vi "Calculate sleeping line length_datumLine.vi"(7 "Datum angle":dbl, 8 "error in (no error)":errorcluster, 9 "Datum origin":cluster{"X":sgl, "Y":sgl} {"Y" format="%.2f"; "X" format="%.2f"}, 10 "Line":T1, 11 "Mouse release \npoint":cluster{"X":dbl, "Y":dbl}) -> (0 "error out":errorcluster, 2 "Angle offset":dbl, 3 "Slanting line\nlength":sgl)   [LabVIEW 2019]
uses:
  <vilib>/vision/NI_Vision_Development_Module.lvlib
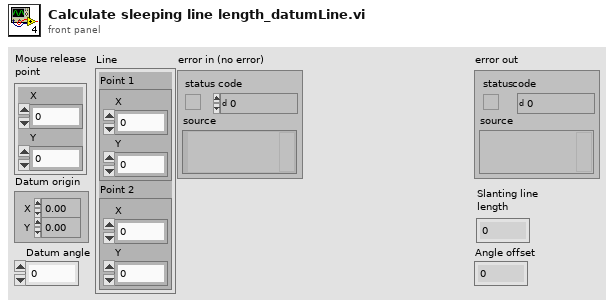
[diagram p1: front panel]
types:
  T1 = cluster{"Point 1":cluster{"X":sgl, "Y":sgl}, "Point 2":cluster{"X":sgl, "Y":sgl}}
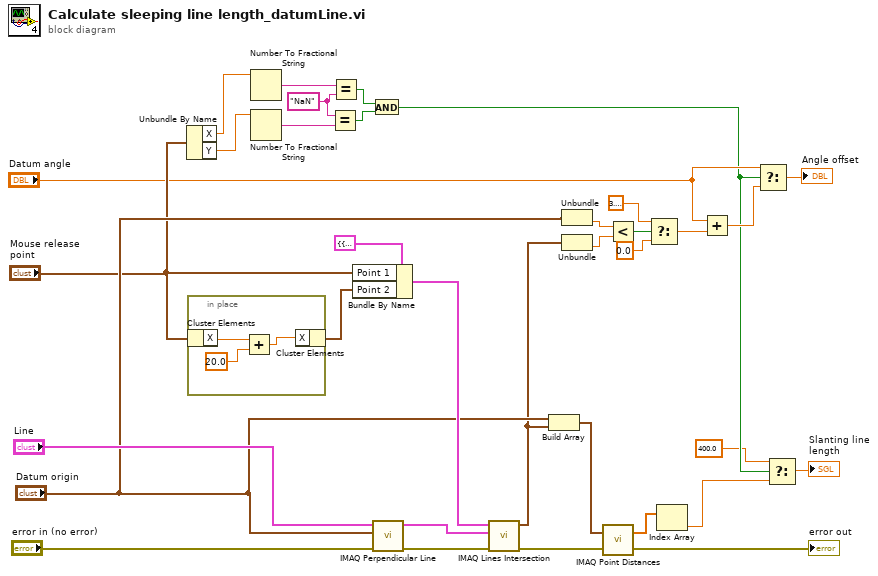
[diagram p0: block diagram]
diagram:
  w10 = "NaN" ("y")
  n1 = Unbundle By Name("Mouse release \npoint") -> ("X"=w14:dbl, "Y"=w13:dbl)
  n2 = in-place {
    n3 = in-place-cluster #1("Mouse release \npoint") -> ("X"=w37:dbl)
    n4 = Add(x=w37, y=20.0) -> (x+y=w35:dbl)
    n5 = in-place-cluster #1("X"=w35) -> (w31:cluster{"X":dbl, "Y":dbl})
  }
  n6 = Number To Fractional String(number=w14) -> (F-format string=w12:string)  [unwired: 3 in]
  n7 = Number To Fractional String(number=w13) -> (F-format string=w11:string)  [unwired: 3 in]
  n8 = Equal?(x=w10, y=w11) -> (x = y?=w8:bool)
  n9 = Equal?(x=w12, y=w10) -> (x = y?=w9:bool)
  n10 = Bundle By Name(cluster=T1 {"Point 1"={"X"=0.0, "Y"=0.0}, "Point 2"={"X"=0.0, "Y"=0.0}} ("Line 1"), "Point 1"="Mouse release \npoint", "Point 2"=w31) -> (w30:T1)
  n11 = And(x=w9, y=w8) -> (x .and. y?=w4:bool)
  n12 = call "IMAQ Perpendicular Line"("error in (no error)"="error in (no error)", "Point"="Datum origin", "Line"="Line") -> ("error out"=w28:errorcluster, "Perpendicular Line"=w29:T1)  [unwired: 6 in, 1 out]
  n13 = call "IMAQ Lines Intersection"("error in (no error)"=w28, "Line 2"=w29, "Line 1"=w30) -> ("error out"=w26:errorcluster, "Intersection Point"=w22:cluster{"X":sgl, "Y":sgl})  [unwired: 6 in, 1 out]
  n14 = Build Array("Datum origin", w22) -> (w27:cluster{"X":sgl, "Y":sgl}[])
  n15 = Unbundle("Datum origin") -> ("Y"=w21:sgl)  [unwired: 1 out]
  n16 = Unbundle(w22) -> ("Y"=w20:sgl)  [unwired: 1 out]
  n17 = call "IMAQ Point Distances"("Points"=w27, "error in (no error)"=w26) -> ("Distances"=w24:sgl[], "error out"=→"error out":errorcluster)  [unwired: 3 in]
  n18 = Less?(x=w21, y=w20) -> (x < y?=w19:bool)
  n19 = Select(t=3.141592653589793, s=w19, f=0.0) -> (s? t:f=w16:dbl)
  n20 = Index Array(array=w24) -> (element=w3:sgl)  [unwired: 1 in]
  n21 = Add(x="Datum angle", y=w16) -> (x+y=w6:dbl)
  n22 = Select(t="Datum angle", s=w4, f=w6) -> (s? t:f=→"Angle offset":dbl)
  n23 = Select(t=sgl 400.0, s=w4, f=w3) -> (s? t:f=→"Slanting line\nlength":sgl)
